vi "set_mixture.vi"() -> (0 "Fuel Mole Fraction":dbl, 1 "Oxidizer Mole Fraction":dbl, 2 "Diluent Mole Fraction":dbl, 3 "Equivalence Ratio":dbl, 4 "Initial Pressure":dbl[unit], 5 "Fuel":string, 6 "Oxidizer":string, 7 "Diluent":string)   [LabVIEW 2018]
panel:
  in  "Initial Pressure":dbl[unit]=101325.0 min=0.0
  in  "Cancel":bool
  in  "Diluent Mole Fraction":dbl min=0.0 max=1.0
  in  "Equivalence Ratio":dbl=1.0 min=0.0
  in  "Diluent":string(combo)="None"
  in  "Oxidizer":string(combo)="N2O"
  in  "Fuel":string(combo)="CH4"
  in  "Done":bool
  in  "Mechanism":string(combo)="gri30.cti"
  # "Set Gas Mixture"
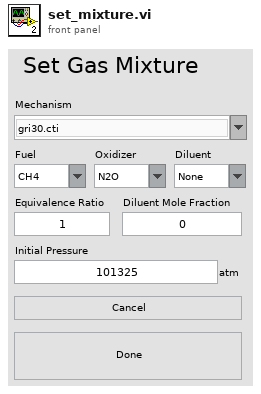
[diagram p1: front panel]
types:
  T1 = enum16{"Always On", "Always Off", "Off While Running"}
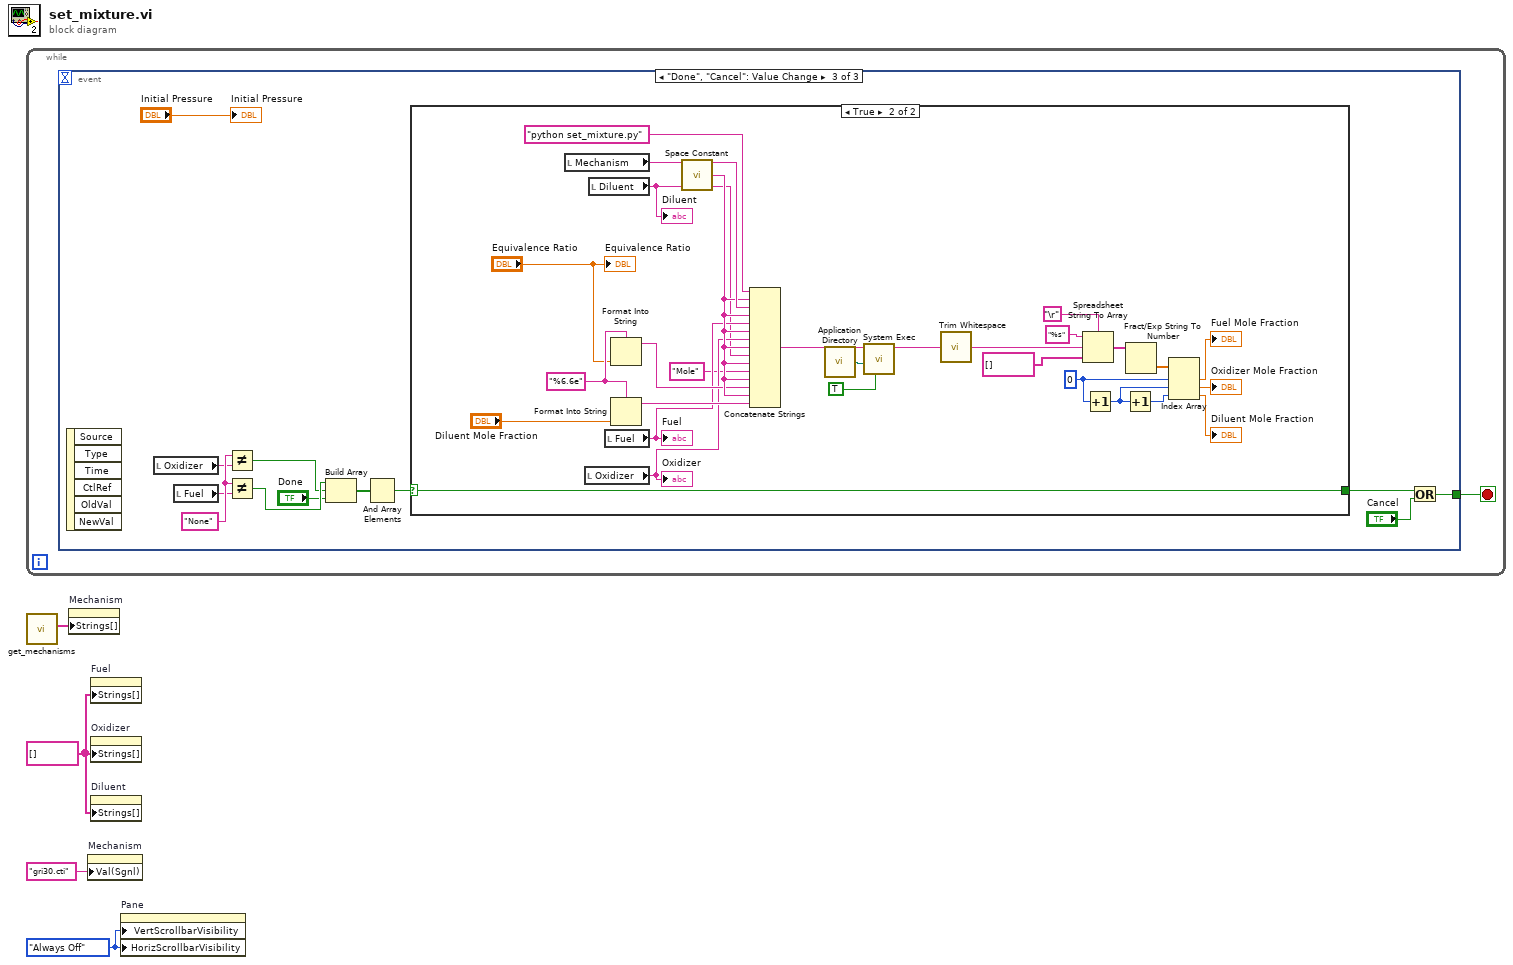
[diagram p0: block diagram]
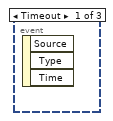
[diagram p2: hidden frame]
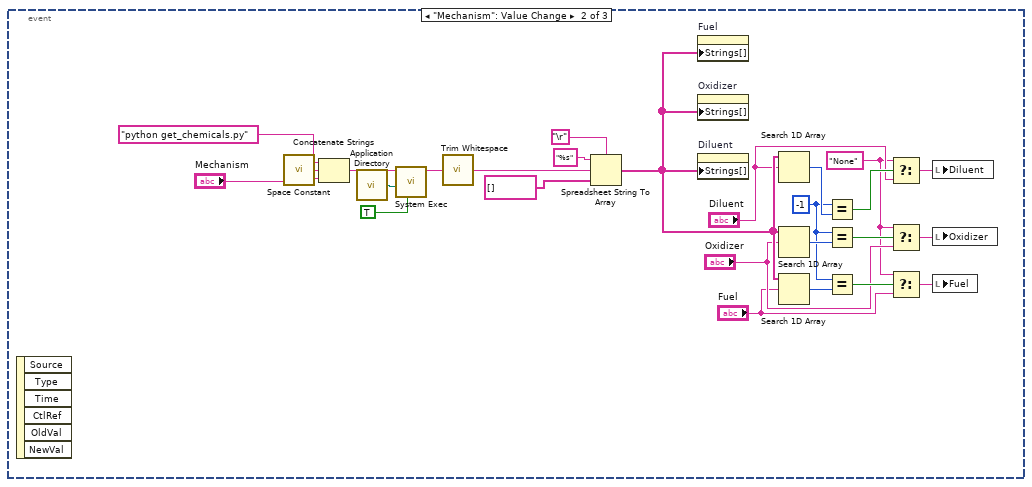
[diagram p3: hidden frame]
diagram:
  w1 = string[] [] ("Strings []")
  w2 = T1."Always Off" ("Vertical Scrollbar Visibility")
  n1 = while {
    stop <- w5 stop-if-true
    n2 = event shown="[2] \"Done\", \"Cancel\": Value Change" {
      selector: _ -> [_ _ _]
      dyn-events: _ -> [_ _ _]
      timeout: _ -> [_ _ _]
      tunnel: [_ _ w34] -> w5
      event Timeout {
        n3 = event-data() -> ()  [unwired: 1 in, 3 out]
      }
      event "Mechanism": Value Change {
        w9 = "None" ("t")
        w16 = -1 ("x")
        n4 = event-data() -> ()  [unwired: 1 in, 6 out]
        n5 = call <vilib>:"Space Constant.vi"() -> ("String"=w30:string)
        n6 = Concatenate Strings("python get_chemicals.py" ("command line"), w30, "Mechanism") -> (w27:string)
        n7 = call <vilib>:"Application Directory.vi"() -> ("Application Directory"=w31:path)
        n8 = call <vilib>:"System Exec.vi"("run minimized? (F)"=TRUE, "working directory"=w31, "command line"=w27) -> ("standard output"=w26:string)  [unwired: 5 in, 3 out]
        n9 = call <vilib>:"Trim Whitespace.vi"("string"=w26) -> ("trimmed string"=w25:string)  [unwired: 1 in]
        n10 = Spreadsheet String To Array(delimiter (Tab)="\r", format string="%s", spreadsheet string=w25, array type (2D Dbl)=string[] []) -> (array=w20:string[])
        n11 = property on="Fuel" class="CmbBox"("Strings[]"=w20) -> ()  [unwired: 2 in, 2 out]
        n12 = property on="Oxidizer" class="CmbBox"("Strings[]"=w20) -> ()  [unwired: 2 in, 2 out]
        n13 = property on="Diluent" class="CmbBox"("Strings[]"=w20) -> ()  [unwired: 2 in, 2 out]
        n14 = Search 1D Array(1D array=w20, element="Diluent") -> (index of element=w17:i32)  [unwired: 1 in]
        n15 = Search 1D Array(1D array=w20, element="Oxidizer") -> (index of element=w18:i32)  [unwired: 1 in]
        n16 = Search 1D Array(1D array=w20, element="Fuel") -> (index of element=w19:i32)  [unwired: 1 in]
        n17 = Equal?(x=w16, y=w17) -> (x = y?=w13:bool)
        n18 = Equal?(x=w16, y=w18) -> (x = y?=w14:bool)
        n19 = Equal?(x=w16, y=w19) -> (x = y?=w15:bool)
        n20 = Select(t=w9, s=w13, f="Diluent") -> (s? t:f=w7:string)
        n21 = Select(t=w9, s=w14, f="Oxidizer") -> (s? t:f=w6:string)
        n22 = Select(t=w9, s=w15, f="Fuel") -> (s? t:f=w8:string)
        n23 = local write "Diluent"(w7) -> ()
        n24 = local write "Oxidizer"(w6) -> ()
        n25 = local write "Fuel"(w8) -> ()
      }
      event "Done", "Cancel": Value Change {
        w39 = "None"
        n26 = event-data() -> ()  [unwired: 1 in, 6 out]
        n27 = local read "Oxidizer"() -> (w38:string)
        n28 = local read "Fuel"() -> (w37:string)
        n29 = Not Equal?(x=w39, y=w38) -> (x != y?=w41:bool)
        n30 = Not Equal?(x=w39, y=w37) -> (x != y?=w42:bool)
        n31 = Build Array(w42, w41, "Done") -> (w43:bool[])
        n32 = And Array Elements(Boolean array=w43) -> (logical AND=w36:bool)
        n33 = case shown="True" w36 {
          selector: w36 -> [w44 w70]
          tunnel: [w44 w70] -> w35
          frame False {
          }
          frame True {
            w56 = 0 ("index")
            w67 = "%6.6e" ("format string")
            n34 = local read "Mechanism"() -> (w72:string)
            n35 = local read "Oxidizer"() -> (w49:string)
            "Oxidizer" <- w49
            n36 = local read "Diluent"() -> (w48:string)
            "Diluent" <- w48
            n37 = local read "Fuel"() -> (w50:string)
            "Fuel" <- w50
            n38 = Format Into String(format string=w67, "Equivalence Ratio") -> (resulting string=w69:string)  [unwired: 2 in, 1 out]
            n39 = Format Into String(format string=w67, "Diluent Mole Fraction") -> (resulting string=w68:string)  [unwired: 2 in, 1 out]
            n40 = call <vilib>:"Space Constant.vi"() -> ("String"=w71:string)
            n41 = Concatenate Strings("python set_mixture.py", w71, w72, w71, w50, w71, w49, w71, w48, w71, "Mole" ("string"), w71, w69, w71, w68) -> (w63:string)
            n42 = call <vilib>:"Application Directory.vi"() -> ("Application Directory"=w66:path)
            n43 = call <vilib>:"System Exec.vi"("run minimized? (F)"=TRUE, "working directory"=w66, "command line"=w63) -> ("standard output"=w65:string)  [unwired: 5 in, 3 out]
            n44 = call <vilib>:"Trim Whitespace.vi"("string"=w65) -> ("trimmed string"=w59:string)  [unwired: 1 in]
            n45 = Spreadsheet String To Array(delimiter (Tab)="\r", format string="%s", spreadsheet string=w59, array type (2D Dbl)=string[] []) -> (array=w58:string[])
            n46 = Increment(x=w56) -> (x+1=w54:i32)
            n47 = Increment(x=w54) -> (x+1=w55:i32)
            n48 = Fract/Exp String To Number(string=w58) -> (number=w57:dbl[])  [unwired: 3 in, 1 out]
            n49 = Index Array(array=w57, index #1=w56, index #2=w54, index #3=w55) -> (element #1=→"Fuel Mole Fraction":dbl, element #2=→"Oxidizer Mole Fraction":dbl, element #3=→"Diluent Mole Fraction":dbl)
            "Equivalence Ratio" <- "Equivalence Ratio"
          }
        }
        n50 = Or(x=w35, y="Cancel") -> (x .or. y?=w34:bool)
        "Initial Pressure" <- "Initial Pressure"
      }
    }
  }
  n51 = call "get_mechanisms.vi"() -> ("Mechanisms"=w3:string[])  [unwired: 11 in]
  n52 = property on="Mechanism" class="CmbBox"("Strings[]"=w3) -> ()  [unwired: 2 in, 2 out]
  n53 = property on="Mechanism" class="CmbBox"("Val(Sgnl)"="gri30.cti") -> ()  [unwired: 2 in, 2 out]
  n54 = property on="Fuel" class="CmbBox"("Strings[]"=w1) -> ()  [unwired: 2 in, 2 out]
  n55 = property on="Oxidizer" class="CmbBox"("Strings[]"=w1) -> ()  [unwired: 2 in, 2 out]
  n56 = property on="Diluent" class="CmbBox"("Strings[]"=w1) -> ()  [unwired: 2 in, 2 out]
  n57 = property on="Pane" class="Pane"("VertScrollbarVisibility"=w2, "HorizScrollbarVisibility"=w2) -> ()  [unwired: 2 in, 2 out]
